vi "Update Position.vi"(8 "Time":dbl, 9 "Speed":dbl, 10 "End Pos":T1, 11 "Start Pos":T1) -> (3 "Current Pos":T1)   [LabVIEW 2019]
doc: "A simple linear move between start and end positions based on the target speed and current time."
uses:
  _2D/Point.ctl
  _2D/2D.lvlib
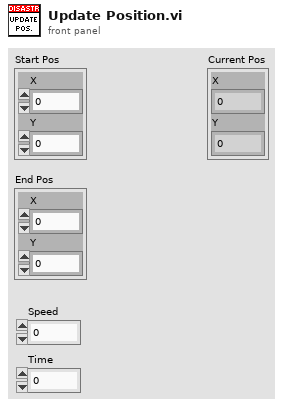
[diagram p1: front panel]
types:
  T1 = typedef "2D.lvlib/Point.ctl" = cluster{"X":i16, "Y":i16}
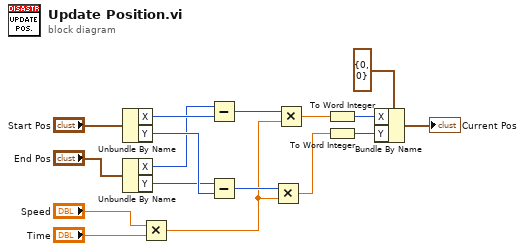
[diagram p0: block diagram]
diagram:
  n1 = Unbundle By Name("Start Pos") -> ("X"=w15:i16, "Y"=w14:i16)
  n2 = Unbundle By Name("End Pos") -> ("X"=w13:i16, "Y"=w12:i16)
  n3 = Multiply(x="Speed", y="Time") -> (x*y=w5:dbl)
  n4 = Subtract(x=w13, y=w15) -> (x-y=w17:i16)
  n5 = Subtract(x=w12, y=w14) -> (x-y=w16:i16)
  n6 = Multiply(x=w16, y=w5) -> (x*y=w10:dbl)
  n7 = Multiply(x=w17, y=w5) -> (x*y=w11:dbl)
  n8 = To Word Integer(number=w11) -> (16bit integer=w3:i16)
  n9 = To Word Integer(number=w10) -> (16bit integer=w4:i16)
  n10 = Bundle By Name(cluster=T1 {"X"=0, "Y"=0} ("input cluster"), "X"=w3, "Y"=w4) -> (→"Current Pos":T1)
